vi "Initialize Deployed Shared Variables.vi"(8 "Error In":errorcluster, 11 "Container refnum in":refnum<k21>="ni.var.psp://localhost") -> (0 "Error Out":errorcluster, 2 "Status":string)   [LabVIEW 2014]
doc: "<B>Copyright</B>: (c) 2015 MHWirth. All rights reserved.\n\n<B>need to improve</B>\n\nThis VI gets all deployed shared variables on the given container, and finds their URL and Type. Later, it opens connection and initializes all the shared variables.\n\nIf the type is not defined, Status will be \"Undefined Type\", and initialization stops at the shared variable index."
uses:
  <vilib>/Utility/error.llb/DialogType.ctl
panel:
  out "URL and Type":string[][](array[string])
  out "Number of Deployed SV":i32
  # "This VI gets the SV information and initializes them."
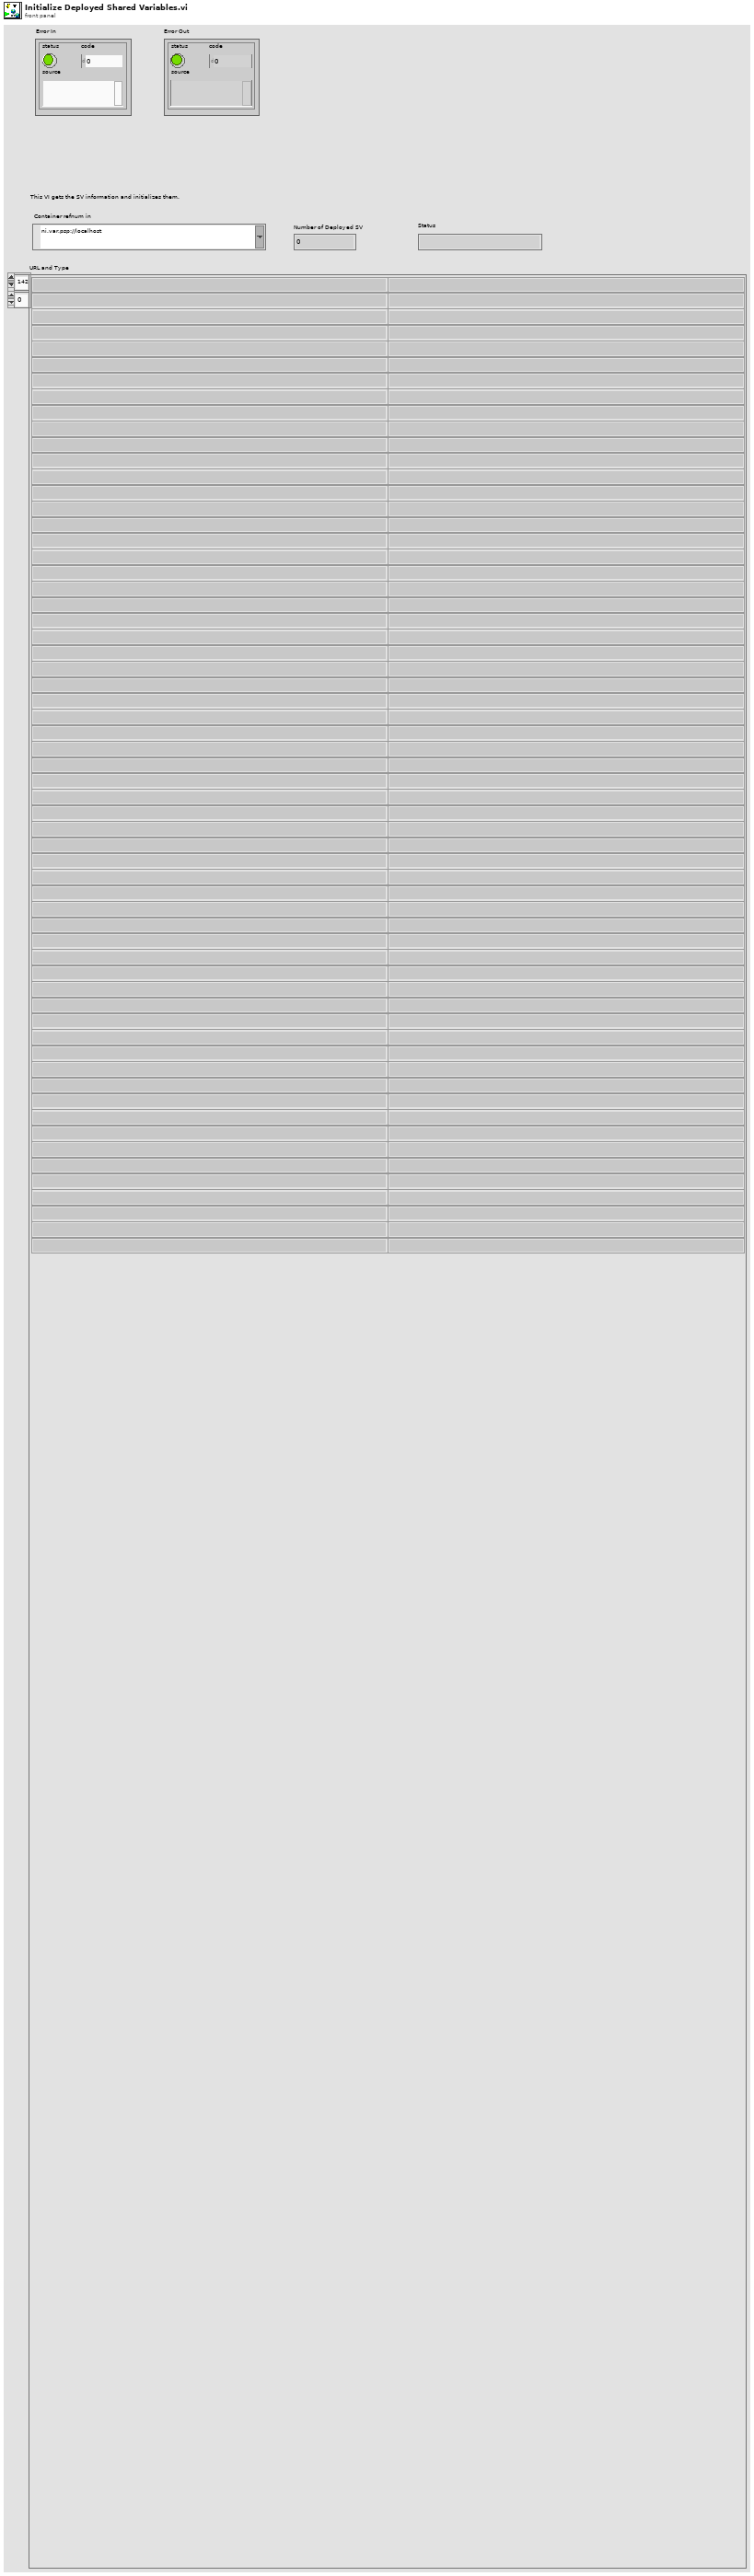
[diagram p1: front panel]
types:
  T1 = typedef "DialogType.ctl" = u16
  T2 = cluster{"Number of Variables":i32, "Variable/Parent Name array":string[][], "URL array":string[], "Type array":string[]}
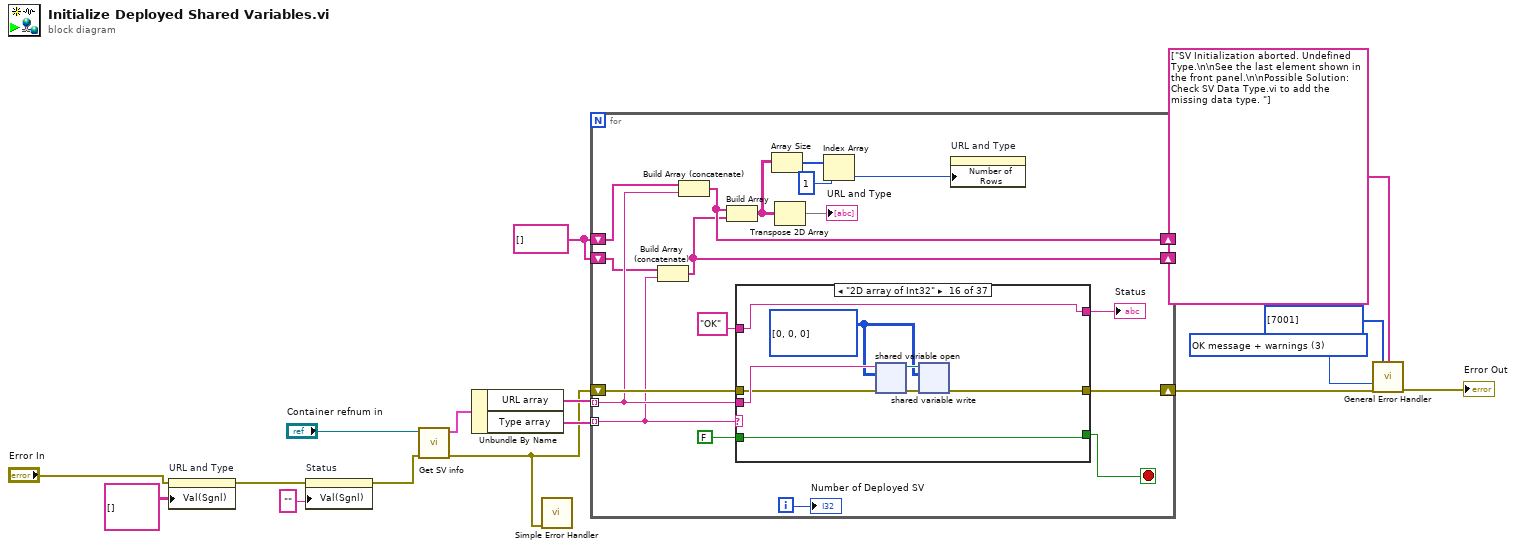
[diagram p0: block diagram]
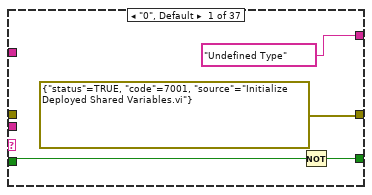
[diagram p2: hidden frame]
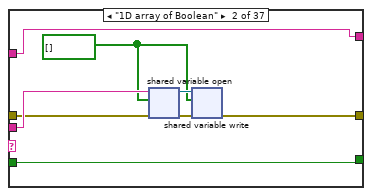
[diagram p3: hidden frame]
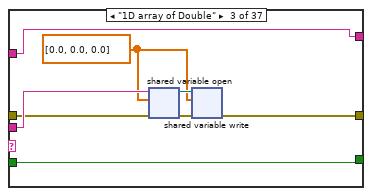
[diagram p4: hidden frame]
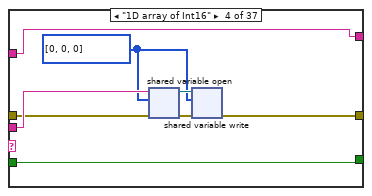
[diagram p5: hidden frame]
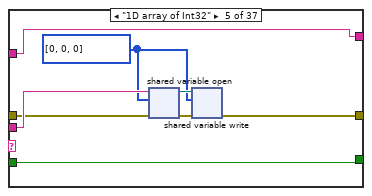
[diagram p6: hidden frame]
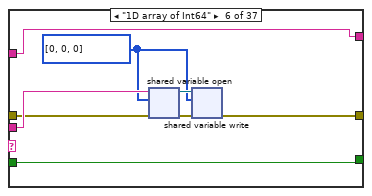
[diagram p7: hidden frame]
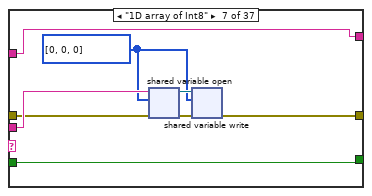
[diagram p8: hidden frame]
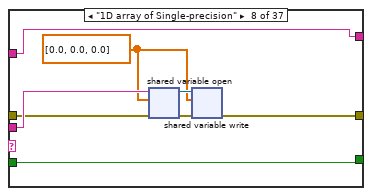
[diagram p9: hidden frame]
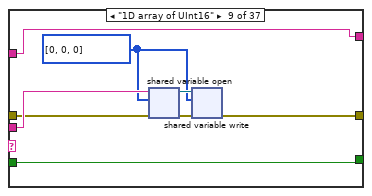
[diagram p10: hidden frame]
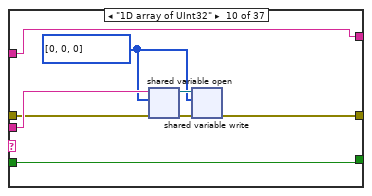
[diagram p11: hidden frame]
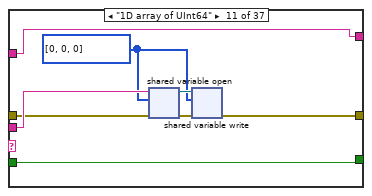
[diagram p12: hidden frame]
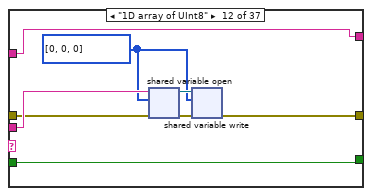
[diagram p13: hidden frame]
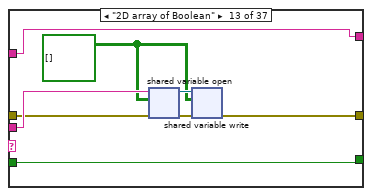
[diagram p14: hidden frame]
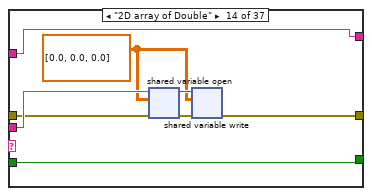
[diagram p15: hidden frame]
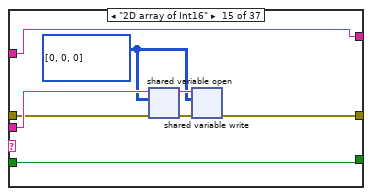
[diagram p16: hidden frame]
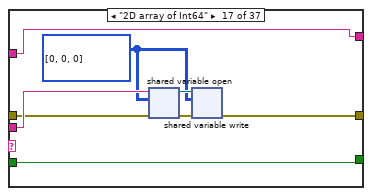
[diagram p17: hidden frame]
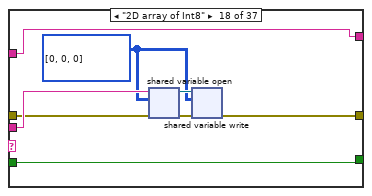
[diagram p18: hidden frame]
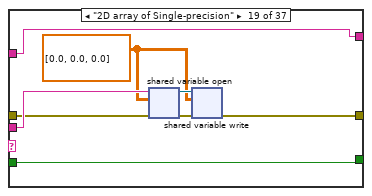
[diagram p19: hidden frame]
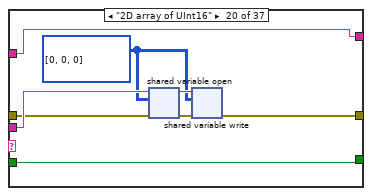
[diagram p20: hidden frame]
diagram:
  w4 = string[] []
  w11 = T1 3 items=["no dialog", "OK message", "continue or stop message", "OK message + warnings", "continue/stop + warnings"] ("type of dialog (OK msg:1)")
  n1 = property on="URL and Type" class="Arr (strict)"(error in="Error In", "Val(Sgnl)"=string[][] [] ("Value (Signaling)")) -> (error out=w6:errorcluster)  [unwired: 1 in, 1 out]
  n2 = property on="Status" class="Str"(error in=w6, "Val(Sgnl)"="" ("Value (Signaling)")) -> (error out=w5:errorcluster)  [unwired: 1 in, 1 out]
  n3 = call "Get SV info.vi"("Error In"=w5, "container refnum in"="Container refnum in") -> ("Error Out"=w3:errorcluster, "Deployed Shared Variable Information"=w16:T2)  [unwired: 7 in, 1 out]
  n4 = Unbundle By Name(w16) -> ("URL array"=w15:string[], "Type array"=w14:string[])
  n5 = call <vilib>:"Simple Error Handler.vi"("error in (no error)"=w3) -> ()  [unwired: 4 in, 5 out]
  n6 = for {
    tunnel: w15 -> [w21] mode=indexing
    tunnel: w14 -> [w19] mode=indexing
    shift-right: [w33] -> w12
    shift-left: w3 -> [w34]
    shift-right: [w18] -> _
    shift-left: w4 -> [w22]
    shift-right: [w17] -> _
    shift-left: w4 -> [w20]
    i -> [w32]
    stop <- w28 stop-if-true
    n7 = Build Array (concatenate)(w20, w19) -> (w17:string[])
    n8 = Build Array (concatenate)(w22, w21) -> (w18:string[])
    n9 = Build Array(w18, w17) -> (w24:string[][])
    n10 = case shown="\"2D array of Int32\"" w19 {
      tunnel: w21 -> [_ w46 w54 w62 w70 w78 w86 w94 w102 w110 w118 w126 w134 w142 w150 w158 w166 w174 w182 w190 w198 w206 w214 w222 w230 w238 w246 w254 w262 w270 w278 w286 w294 w302 w310 w318 w326]
      tunnel: w34 -> [_ w43 w51 w59 w67 w75 w83 w91 w99 w107 w115 w123 w131 w139 w147 w155 w163 w171 w179 w187 w195 w203 w211 w219 w228 w235 w243 w251 w259 w267 w275 w283 w291 w299 w307 w315 w323]
      tunnel: [errorcluster {"status"=TRUE, "code"=7001, "source"="Initialize Deployed Shared Variables.vi"} ("error constant") w41 w49 w57 w65 w73 w81 w89 w97 w105 w113 w121 w129 w137 w145 w153 w161 w169 w177 w185 w193 w201 w209 w217 w226 w233 w241 w249 w257 w265 w273 w281 w289 w297 w305 w313 w321] -> w33
      tunnel: ["Undefined Type" w40 w48 w56 w64 w72 w80 w88 w96 w104 w112 w120 w128 w136 w144 w152 w160 w168 w176 w184 w192 w200 w208 w216 w225 w232 w240 w248 w256 w264 w272 w280 w288 w296 w304 w312 w320] -> w31
      tunnel: "OK" -> [_ w40 w48 w56 w64 w72 w80 w88 w96 w104 w112 w120 w128 w136 w144 w152 w160 w168 w176 w184 w192 w200 w208 w216 w225 w232 w240 w248 w256 w264 w272 w280 w288 w296 w304 w312 w320]
      tunnel: FALSE -> [w37 w39 w47 w55 w63 w71 w79 w87 w95 w103 w111 w119 w127 w135 w143 w151 w159 w167 w175 w183 w191 w199 w207 w215 w224 w231 w239 w247 w255 w263 w271 w279 w287 w295 w303 w311 w319]
      tunnel: [w36 w39 w47 w55 w63 w71 w79 w87 w95 w103 w111 w119 w127 w135 w143 w151 w159 w167 w175 w183 w191 w199 w207 w215 w224 w231 w239 w247 w255 w263 w271 w279 w287 w295 w303 w311 w319] -> w28
      frame "0", Default {
        n11 = Not(x=w37) -> (.not. x?=w36:bool)
      }
      frame "1D array of Boolean" {
        w44 = bool[] []
        n12 = shared-variable-open(w46, w43, w44) -> (w45:refnum<k21>, w42:errorcluster)  [unwired: 1 in]
        n13 = shared-variable-write(w45, w42, w44) -> (w41:errorcluster)  [unwired: 1 out]
      }
      frame "1D array of Double" {
        w52 = dbl[] [0.0, 0.0, 0.0]
        n14 = shared-variable-open(w54, w51, w52) -> (w53:refnum<k21>, w50:errorcluster)  [unwired: 1 in]
        n15 = shared-variable-write(w53, w50, w52) -> (w49:errorcluster)  [unwired: 1 out]
      }
      frame "1D array of Int16" {
        w60 = i16[] [0, 0, 0]
        n16 = shared-variable-open(w62, w59, w60) -> (w61:refnum<k21>, w58:errorcluster)  [unwired: 1 in]
        n17 = shared-variable-write(w61, w58, w60) -> (w57:errorcluster)  [unwired: 1 out]
      }
      frame "1D array of Int32" {
        w68 = i32[] [0, 0, 0]
        n18 = shared-variable-open(w70, w67, w68) -> (w69:refnum<k21>, w66:errorcluster)  [unwired: 1 in]
        n19 = shared-variable-write(w69, w66, w68) -> (w65:errorcluster)  [unwired: 1 out]
      }
      frame "1D array of Int64" {
        w76 = i64[] [0, 0, 0]
        n20 = shared-variable-open(w78, w75, w76) -> (w77:refnum<k21>, w74:errorcluster)  [unwired: 1 in]
        n21 = shared-variable-write(w77, w74, w76) -> (w73:errorcluster)  [unwired: 1 out]
      }
      frame "1D array of Int8" {
        w84 = i8[] [0, 0, 0]
        n22 = shared-variable-open(w86, w83, w84) -> (w85:refnum<k21>, w82:errorcluster)  [unwired: 1 in]
        n23 = shared-variable-write(w85, w82, w84) -> (w81:errorcluster)  [unwired: 1 out]
      }
      frame "1D array of Single-precision" {
        w92 = sgl[] [0.0, 0.0, 0.0]
        n24 = shared-variable-open(w94, w91, w92) -> (w93:refnum<k21>, w90:errorcluster)  [unwired: 1 in]
        n25 = shared-variable-write(w93, w90, w92) -> (w89:errorcluster)  [unwired: 1 out]
      }
      frame "1D array of UInt16" {
        w100 = u16[] [0, 0, 0]
        n26 = shared-variable-open(w102, w99, w100) -> (w101:refnum<k21>, w98:errorcluster)  [unwired: 1 in]
        n27 = shared-variable-write(w101, w98, w100) -> (w97:errorcluster)  [unwired: 1 out]
      }
      frame "1D array of UInt32" {
        w108 = u32[] [0, 0, 0]
        n28 = shared-variable-open(w110, w107, w108) -> (w109:refnum<k21>, w106:errorcluster)  [unwired: 1 in]
        n29 = shared-variable-write(w109, w106, w108) -> (w105:errorcluster)  [unwired: 1 out]
      }
      frame "1D array of UInt64" {
        w116 = u64[] [0, 0, 0]
        n30 = shared-variable-open(w118, w115, w116) -> (w117:refnum<k21>, w114:errorcluster)  [unwired: 1 in]
        n31 = shared-variable-write(w117, w114, w116) -> (w113:errorcluster)  [unwired: 1 out]
      }
      frame "1D array of UInt8" {
        w124 = u8[] [0, 0, 0]
        n32 = shared-variable-open(w126, w123, w124) -> (w125:refnum<k21>, w122:errorcluster)  [unwired: 1 in]
        n33 = shared-variable-write(w125, w122, w124) -> (w121:errorcluster)  [unwired: 1 out]
      }
      frame "2D array of Boolean" {
        w132 = bool[][] []
        n34 = shared-variable-open(w134, w131, w132) -> (w133:refnum<k21>, w130:errorcluster)  [unwired: 1 in]
        n35 = shared-variable-write(w133, w130, w132) -> (w129:errorcluster)  [unwired: 1 out]
      }
      frame "2D array of Double" {
        w140 = dbl[][] [[0.0, 0.0, 0.0]]
        n36 = shared-variable-open(w142, w139, w140) -> (w141:refnum<k21>, w138:errorcluster)  [unwired: 1 in]
        n37 = shared-variable-write(w141, w138, w140) -> (w137:errorcluster)  [unwired: 1 out]
      }
      frame "2D array of Int16" {
        w148 = i16[][] [[0, 0, 0]]
        n38 = shared-variable-open(w150, w147, w148) -> (w149:refnum<k21>, w146:errorcluster)  [unwired: 1 in]
        n39 = shared-variable-write(w149, w146, w148) -> (w145:errorcluster)  [unwired: 1 out]
      }
      frame "2D array of Int32" {
        w156 = i32[][] [[0, 0, 0]]
        n40 = shared-variable-open(w158, w155, w156) -> (w157:refnum<k21>, w154:errorcluster)  [unwired: 1 in]
        n41 = shared-variable-write(w157, w154, w156) -> (w153:errorcluster)  [unwired: 1 out]
      }
      frame "2D array of Int64" {
        w164 = i64[][] [[0, 0, 0]]
        n42 = shared-variable-open(w166, w163, w164) -> (w165:refnum<k21>, w162:errorcluster)  [unwired: 1 in]
        n43 = shared-variable-write(w165, w162, w164) -> (w161:errorcluster)  [unwired: 1 out]
      }
      frame "2D array of Int8" {
        w172 = i8[][] [[0, 0, 0]]
        n44 = shared-variable-open(w174, w171, w172) -> (w173:refnum<k21>, w170:errorcluster)  [unwired: 1 in]
        n45 = shared-variable-write(w173, w170, w172) -> (w169:errorcluster)  [unwired: 1 out]
      }
      frame "2D array of Single-precision" {
        w180 = sgl[][] [[0.0, 0.0, 0.0]]
        n46 = shared-variable-open(w182, w179, w180) -> (w181:refnum<k21>, w178:errorcluster)  [unwired: 1 in]
        n47 = shared-variable-write(w181, w178, w180) -> (w177:errorcluster)  [unwired: 1 out]
      }
      frame "2D array of UInt16" {
        w188 = u16[][] [[0, 0, 0]]
        n48 = shared-variable-open(w190, w187, w188) -> (w189:refnum<k21>, w186:errorcluster)  [unwired: 1 in]
        n49 = shared-variable-write(w189, w186, w188) -> (w185:errorcluster)  [unwired: 1 out]
      }
      frame "2D array of UInt32" {
        w196 = u32[][] [[0, 0, 0]]
        n50 = shared-variable-open(w198, w195, w196) -> (w197:refnum<k21>, w194:errorcluster)  [unwired: 1 in]
        n51 = shared-variable-write(w197, w194, w196) -> (w193:errorcluster)  [unwired: 1 out]
      }
      frame "2D array of UInt64" {
        w204 = u64[][] [[0, 0, 0]]
        n52 = shared-variable-open(w206, w203, w204) -> (w205:refnum<k21>, w202:errorcluster)  [unwired: 1 in]
        n53 = shared-variable-write(w205, w202, w204) -> (w201:errorcluster)  [unwired: 1 out]
      }
      frame "2D array of UInt8" {
        w212 = u8[][] [[0, 0, 0]]
        n54 = shared-variable-open(w214, w211, w212) -> (w213:refnum<k21>, w210:errorcluster)  [unwired: 1 in]
        n55 = shared-variable-write(w213, w210, w212) -> (w209:errorcluster)  [unwired: 1 out]
      }
      frame "Boolean" {
        w220 = FALSE
        n56 = shared-variable-open(w222, w219, w220) -> (w221:refnum<k21>, w218:errorcluster)  [unwired: 1 in]
        n57 = shared-variable-write(w221, w218, w220) -> (w217:errorcluster)  [unwired: 1 out]
      }
      frame "String" {
        w223 = "dummy"
        n58 = shared-variable-open(w230, w228, w223) -> (w229:refnum<k21>, w227:errorcluster)  [unwired: 1 in]
        n59 = shared-variable-write(w229, w227, w223) -> (w226:errorcluster)  [unwired: 1 out]
      }
      frame "Double" {
        w236 = 0.0
        n60 = shared-variable-open(w238, w235, w236) -> (w237:refnum<k21>, w234:errorcluster)  [unwired: 1 in]
        n61 = shared-variable-write(w237, w234, w236) -> (w233:errorcluster)  [unwired: 1 out]
      }
      frame "Fixed Point - signed" {
        w244 = fxp<+/-,32,16> 0.0
        n62 = shared-variable-open(w246, w243, w244) -> (w245:refnum<k21>, w242:errorcluster)  [unwired: 1 in]
        n63 = shared-variable-write(w245, w242, w244) -> (w241:errorcluster)  [unwired: 1 out]
      }
      frame "Fixed Point - unsigned" {
        w252 = fxp<+,32,16> 0.0
        n64 = shared-variable-open(w254, w251, w252) -> (w253:refnum<k21>, w250:errorcluster)  [unwired: 1 in]
        n65 = shared-variable-write(w253, w250, w252) -> (w249:errorcluster)  [unwired: 1 out]
      }
      frame "Int16" {
        w260 = i16 0
        n66 = shared-variable-open(w262, w259, w260) -> (w261:refnum<k21>, w258:errorcluster)  [unwired: 1 in]
        n67 = shared-variable-write(w261, w258, w260) -> (w257:errorcluster)  [unwired: 1 out]
      }
      frame "Int32" {
        w268 = 0
        n68 = shared-variable-open(w270, w267, w268) -> (w269:refnum<k21>, w266:errorcluster)  [unwired: 1 in]
        n69 = shared-variable-write(w269, w266, w268) -> (w265:errorcluster)  [unwired: 1 out]
      }
      frame "Int64" {
        w276 = i64 0
        n70 = shared-variable-open(w278, w275, w276) -> (w277:refnum<k21>, w274:errorcluster)  [unwired: 1 in]
        n71 = shared-variable-write(w277, w274, w276) -> (w273:errorcluster)  [unwired: 1 out]
      }
      frame "Int8" {
        w284 = i8 0
        n72 = shared-variable-open(w286, w283, w284) -> (w285:refnum<k21>, w282:errorcluster)  [unwired: 1 in]
        n73 = shared-variable-write(w285, w282, w284) -> (w281:errorcluster)  [unwired: 1 out]
      }
      frame "Single-precision" {
        w292 = sgl 0.0
        n74 = shared-variable-open(w294, w291, w292) -> (w293:refnum<k21>, w290:errorcluster)  [unwired: 1 in]
        n75 = shared-variable-write(w293, w290, w292) -> (w289:errorcluster)  [unwired: 1 out]
      }
      frame "UInt16" {
        w300 = u16 0
        n76 = shared-variable-open(w302, w299, w300) -> (w301:refnum<k21>, w298:errorcluster)  [unwired: 1 in]
        n77 = shared-variable-write(w301, w298, w300) -> (w297:errorcluster)  [unwired: 1 out]
      }
      frame "UInt32" {
        w308 = u32 0
        n78 = shared-variable-open(w310, w307, w308) -> (w309:refnum<k21>, w306:errorcluster)  [unwired: 1 in]
        n79 = shared-variable-write(w309, w306, w308) -> (w305:errorcluster)  [unwired: 1 out]
      }
      frame "UInt64" {
        w316 = u64 0
        n80 = shared-variable-open(w318, w315, w316) -> (w317:refnum<k21>, w314:errorcluster)  [unwired: 1 in]
        n81 = shared-variable-write(w317, w314, w316) -> (w313:errorcluster)  [unwired: 1 out]
      }
      frame "UInt8" {
        w324 = u8 0
        n82 = shared-variable-open(w326, w323, w324) -> (w325:refnum<k21>, w322:errorcluster)  [unwired: 1 in]
        n83 = shared-variable-write(w325, w322, w324) -> (w321:errorcluster)  [unwired: 1 out]
      }
    }
    "Status" <- w31
    n84 = Array Size(array=w24) -> (size(s)=w25:i32[])
    n85 = Transpose 2D Array(2D array=w24) -> (transposed array=→"URL and Type":string[][])
    n86 = Index Array(array=w25, index=1) -> (element=w26:i32)
    n87 = property on="URL and Type" class="Arr (strict)"("Number of Rows"=w26) -> ()  [unwired: 2 in, 2 out]
    "Number of Deployed SV" <- w32
  }
  n88 = call <vilib>:"General Error Handler.vi"("[user-defined codes]"=i32[] [7001], "[user-defined descriptions]"=string[] ["SV Initialization aborted. Undefined Type.\n\nSee the last element shown in the front panel.\n\nPossible Solution: Check SV Data Type.vi to add the missing data type. "], "type of dialog (OK msg:1)"=w11, "error in (no error)"=w12) -> ("error out"=→"Error Out":errorcluster)  [unwired: 7 in, 4 out]
